vi "LVDT-test_local.vi"() -> ()   [LabVIEW 2011]
uses:
  <vilib>/Analysis/2dsp.llb/Real FFT.vi
  <vilib>/Analysis/NI_AALPro.lvlib
panel:
  in  "FTT-samples":i32=1000
  in  "Level":dbl
  in  "Frequency":dbl
  in  "Remove DC":bool
  in  "DC Level":bool
  in  "Sinus":bool
  in  "Random":bool
  out "size(s)":i32
  in  "stop":bool
  out "FFT graph":dbl[](graph)
  out "Averaged Data":dbl[](array[numeric])
  out "FFT {X}":dbl[](array[numeric])
  out "Time Series":cluster{dbl, dbl, dbl[]}(graph)
  in  "Slide":dbl(slide) scale=0.0..25.0
  in  "n_sample":i32
  out "Complete Data":dbl[](array[numeric])
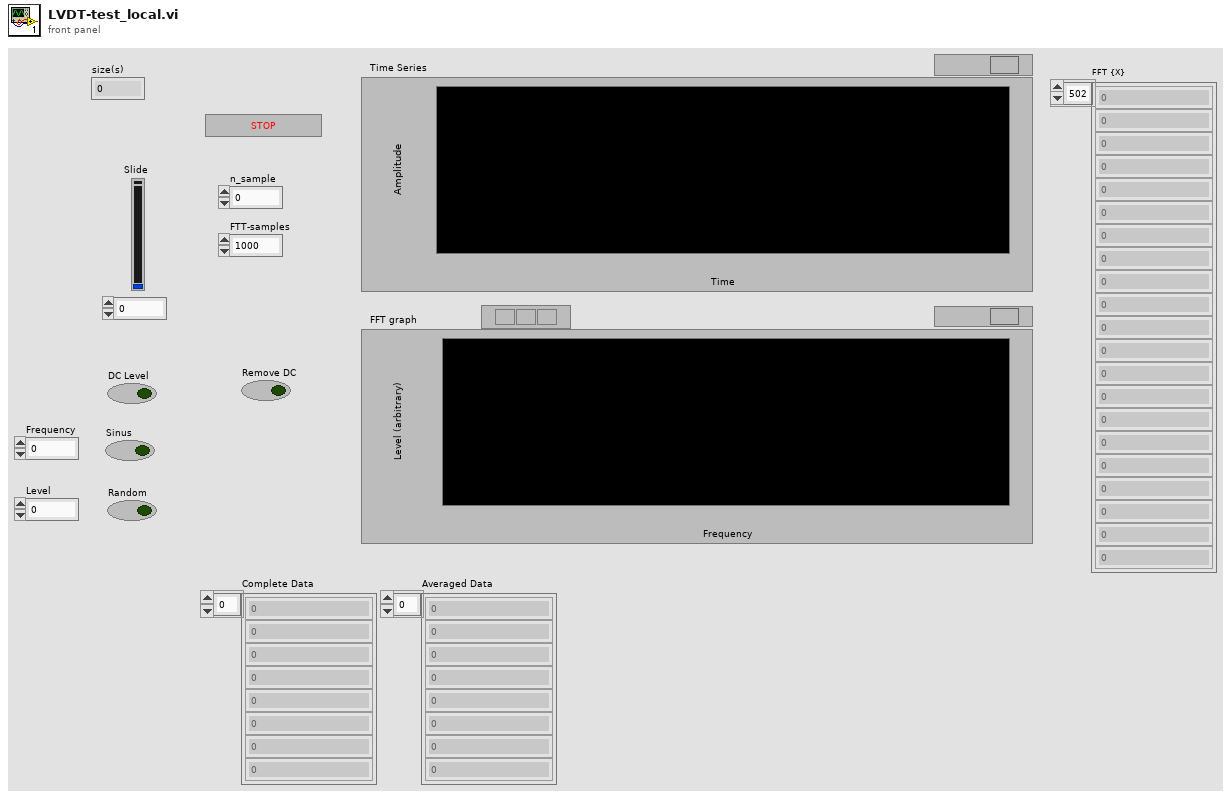
[diagram p1: front panel]
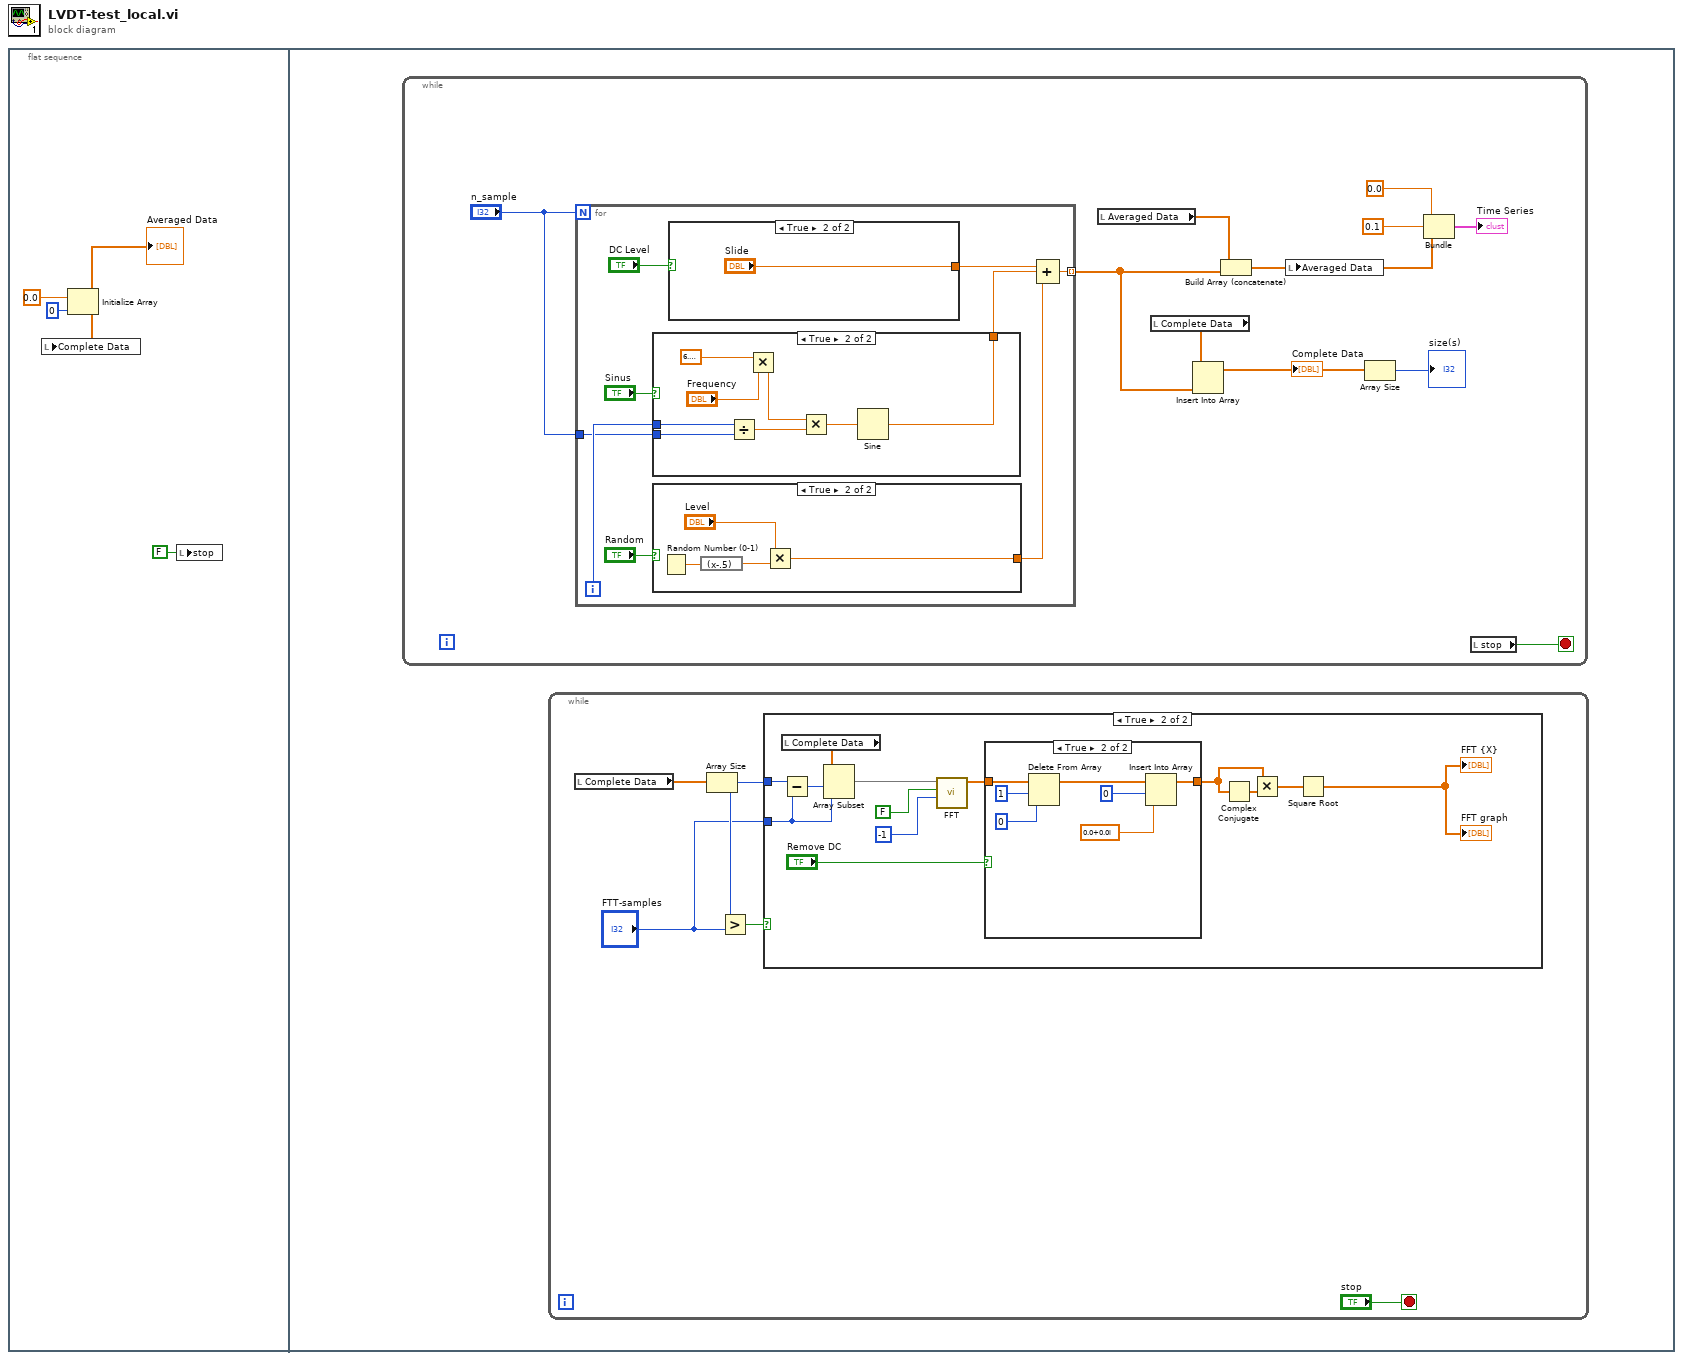
[diagram p0: block diagram]
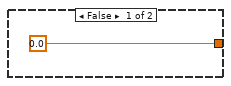
[diagram p2: hidden frame]
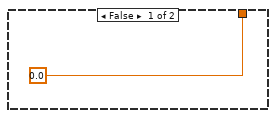
[diagram p3: hidden frame]
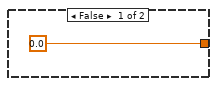
[diagram p4: hidden frame]
diagram:
  n1 = flat-sequence {
    frame #0 {
      n2 = Initialize Array(0.0, 0 ("dimension size")) -> (w2:dbl[])
      "Averaged Data" <- w2
      n3 = local write "Complete Data"(w2) -> ()
      n4 = local write "stop"(FALSE ("stop")) -> ()
    }
    frame #1 {
      n5 = while {
        stop <- w9 stop-if-true
        n6 = for {
          N: "n_sample" -> [_]
          tunnel: [w24] -> w5 mode=indexing
          tunnel: "n_sample" -> [w19]
          i -> [w20]
          n7 = case shown="True" "Sinus" {
            tunnel: [0.0 ("number: 0 to 1") w35] -> w22
            tunnel: w20 -> [_ w34]
            tunnel: w19 -> [_ w33]
            frame False {
            }
            frame True {
              n8 = Divide(x=w34, y=w33) -> (x/y=w32:dbl)
              n9 = Multiply(x=6.283185307179586, y="Frequency") -> (x*y=w30:dbl)
              n10 = Multiply(x=w30, y=w32) -> (x*y=w31:dbl)
              n11 = Sine(x=w31) -> (sin(x)=w35:dbl)
            }
          }
          n12 = case shown="True" "Random" {
            tunnel: [0.0 ("number: 0 to 1") w38] -> w23
            frame False {
            }
            frame True {
              n13 = Random Number (0-1)() -> (number: 0 to 1=w40:dbl)
              n14 = expression code="(x-.5)"(w40) -> (w39:dbl)
              n15 = Multiply(x="Level", y=w39) -> (x*y=w38:dbl)
            }
          }
          n16 = case shown="True" "DC Level" {
            tunnel: [0.0 ("number: 0 to 1") "Slide"] -> w21
            frame False {
            }
            frame True {
            }
          }
          n17 = Compound Arithmetic op=ADD(w21, w22, w23) -> (w24:dbl)
        }
        n18 = local read "Averaged Data"() -> (w14:dbl[])
        n19 = local read "Complete Data"() -> (w15:dbl[])
        n20 = Insert Into Array(array=w15, new element=w5) -> (w8:dbl[])  [unwired: 1 in]
        "Complete Data" <- w8
        n21 = Build Array (concatenate)(w14, w5) -> (w13:dbl[])
        n22 = local write "Averaged Data"(w13) -> ()
        n23 = Array Size(array=w8) -> (size(s)=→"size(s)":i32)
        n24 = Bundle(0.0, 0.1, w13) -> (→"Time Series":cluster{dbl, dbl, dbl[]})  [unwired: 1 in]
        n25 = local read "stop"() -> (w9:bool)
      }
      n26 = while {
        stop <- "stop" stop-if-true
        n27 = local read "Complete Data"() -> (w44:dbl[])
        n28 = Array Size(array=w44) -> (size(s)=w42:i32)
        n29 = Greater?(x=w42, y="FTT-samples") -> (0:w43:bool)
        n30 = case shown="True" w43 {
          tunnel: "FTT-samples" -> [_ w52]
          tunnel: w42 -> [_ w54]
          frame False {
          }
          frame True {
            n31 = local read "Complete Data"() -> (w56:dbl[])
            n32 = Subtract(x=w54, y=w52) -> (x-y=w53:i32)
            n33 = Array Subset(array=w56, index=w53, length=w52) -> (w55:dbl[])
            n34 = call-poly <vilib>:"FFT.vi"("FFT size"=-1, "shift?"=FALSE, "X"=w55) -> ("FFT {X}"=w50:cdb[])  [unwired: 7 in, 1 out]
            n35 = case shown="True" "Remove DC" {
              tunnel: w50 -> [w59 w66]
              tunnel: [w59 w62] -> w49
              frame False {
              }
              frame True {
                n36 = Delete From Array(array=w66, length=1, index=0 ("FFT size")) -> (array with subset deleted=w63:cdb[])  [unwired: 1 out]
                n37 = Insert Into Array(array=w63, index=0 ("FFT size"), new element=cdb 0.0+0.0i ("new element/subarray")) -> (w62:cdb[])
              }
            }
            n38 = Complex Conjugate(1:w49) -> (0:w51:cdb[])
            n39 = Multiply(x=w49, y=w51) -> (x*y=w47:cdb[])
            n40 = Square Root(x=w47) -> (sqrt(x)=→"FFT {X}" →"FFT graph":cdb[])
          }
        }
      }
    }
  }
